vi "SRS865A_api -- V2.vi"(4 "Oscillator (0)":u16, 6 "delay-circle(msec)":i64, 7 "MFLI frontend action":T1=enum."open", 8 "Error In":errorcluster, 10 "Freq IN (Hz)":dbl=40000.0 format="%#_13g", 11 "SRS865 visa":refnum<visa-resource-name>="GPIB0::4::INSTR") -> (0 "Error Out":errorcluster={"status"=TRUE, "code"=-1074003951, "source"="Stanford Research SR865.lvlib:Initialize.vi<ERR>\nThe ID Query failed.  This may mean that you selected the wrong instrument or your instrument did not respond.  You may also be using a model that is not officially supported by this driver.  If you are sure that you have selected the correct instrument and it is responding, try disabling the ID Query.\n\n\n<b>Complete call chain:</b>\r\n     Stanford Research SR865.lvlib:Initialize.vi\r\n     SRS865A_api -- V2.vi\r\n     SRS865A--reader--V2.vi"}, 1 "z out (V)":cdb, 2 "Freq out (Hz)":dbl format="%#_13g", 3 "SRS865 visa OUT":refnum<visa-resource-name>)   [LabVIEW 2017]
uses:
  MFLI frontend action.ctl
  <instrlib>/Zurich Instruments LabOne/Zurich Instruments LabOne.lvlib
  <instrlib>/Stanford Research SR865/Stanford Research SR865.lvlib
panel:
  out "output 1":i32
  in  "timeconstant (s)":dbl=0.006
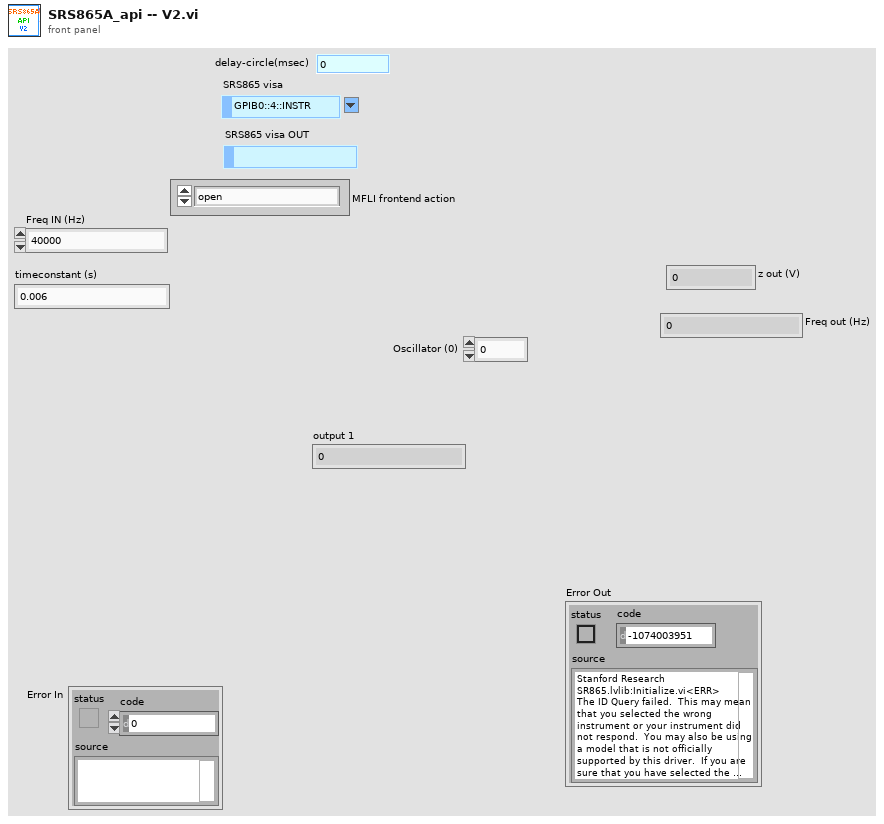
[diagram p1: front panel]
types:
  T1 = typedef "MFLI frontend action.ctl" = enum16{"read", "writeread", "open", "close", "write"}
  T2 = typedef "Zurich Instruments LabOne.lvlib/ziTypeHandle.ctl" = cluster{"handleValid":bool, "Conn":u64, "Path Prefix":string, "Handle":u64, "Connected":bool, "Clockbase(s)":dbl}
  T3 = cluster{"Timestamps (ticks)":u64, "X (Vrms)":dbl, "Y (Vrms)":dbl, "Osc Phase (deg)":dbl, "Freq (Hz)":dbl, "DIO":u32, "AuxIn0 (V)":dbl, "AuxIn1 (V)":dbl}
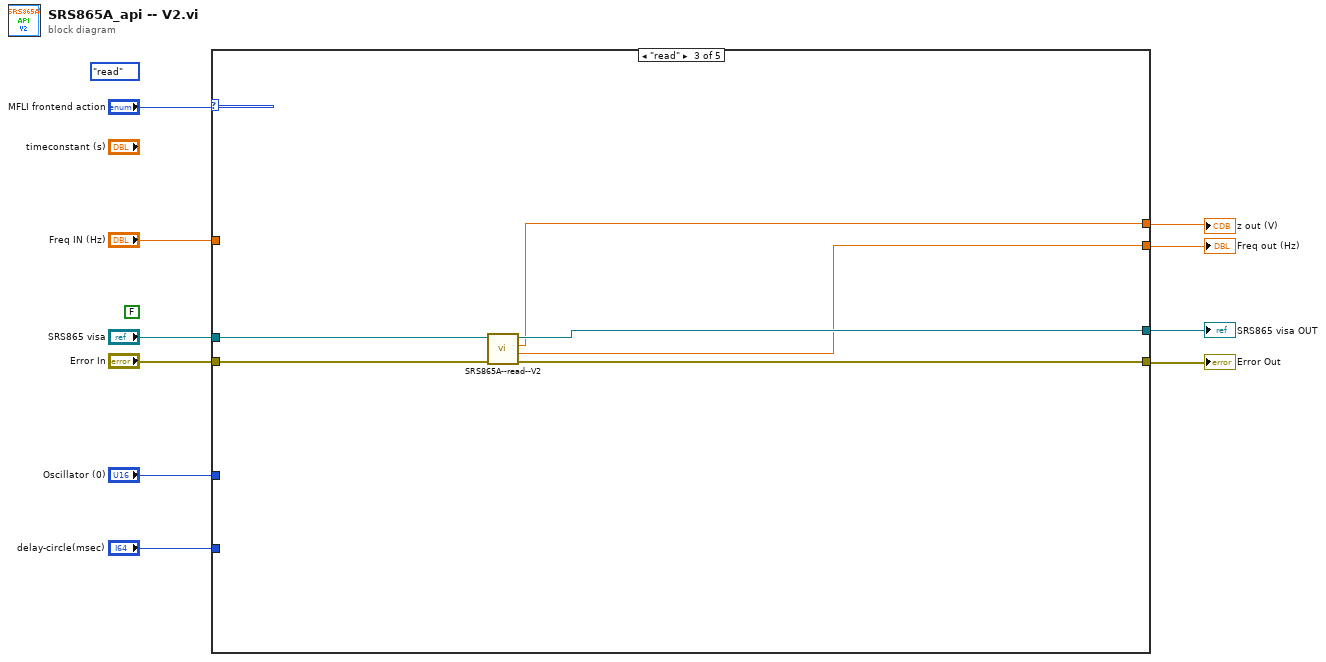
[diagram p0: block diagram]
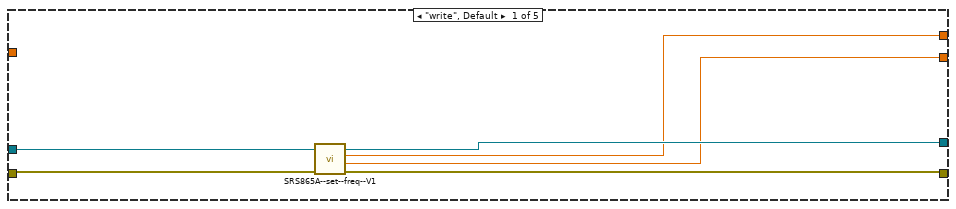
[diagram p2: hidden frame]
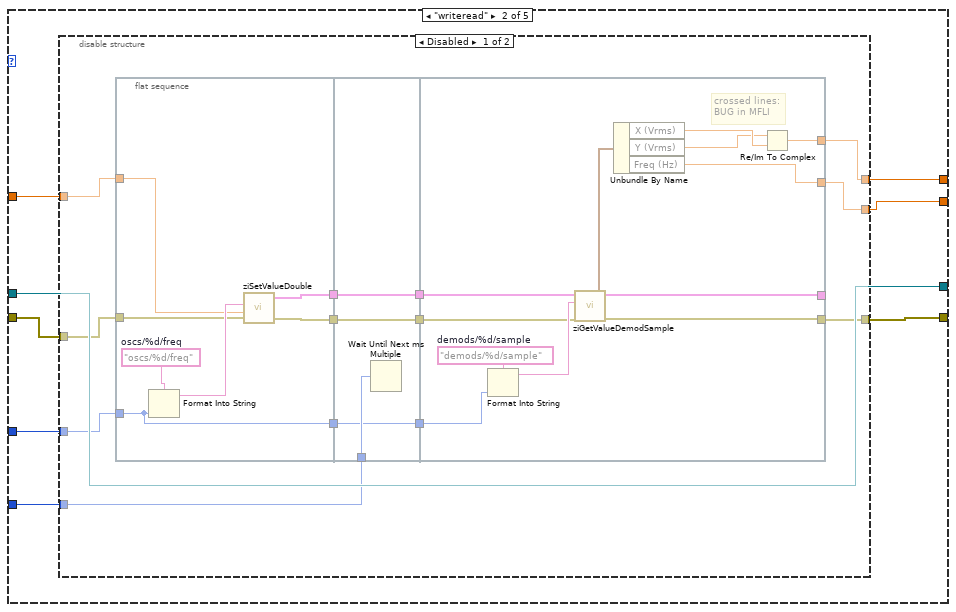
[diagram p3: hidden frame]
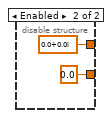
[diagram p4: hidden frame]
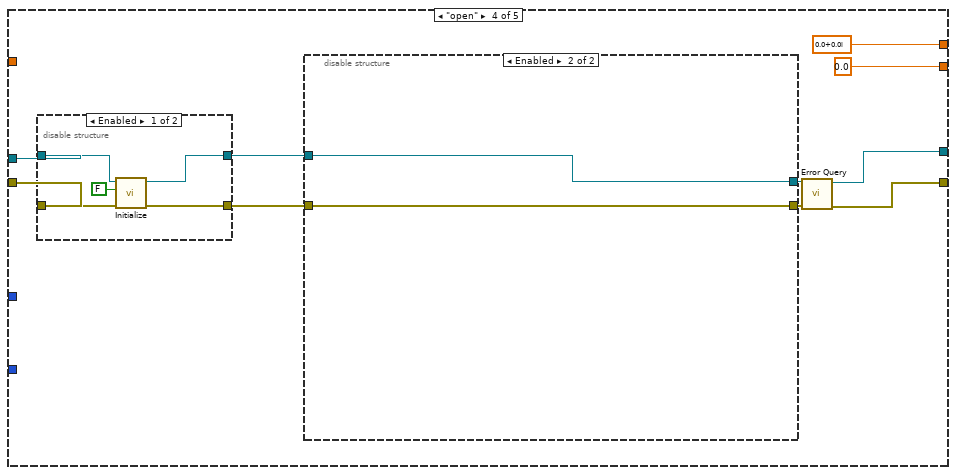
[diagram p5: hidden frame]
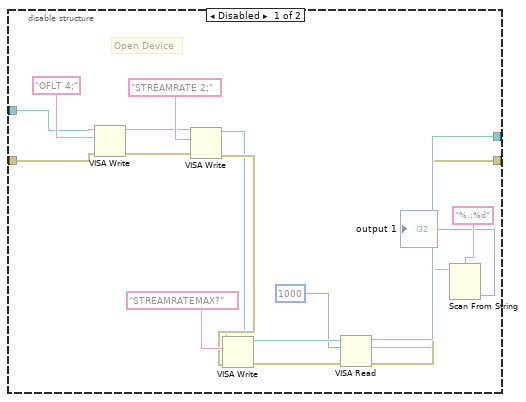
[diagram p6: hidden frame]
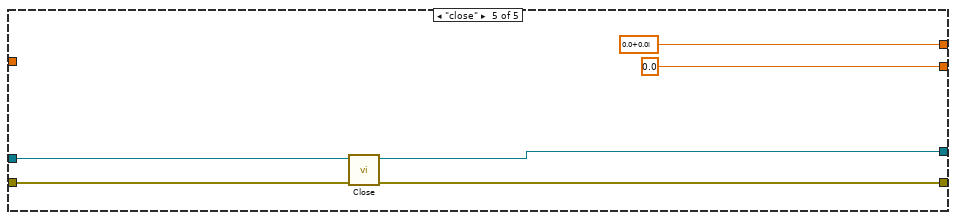
[diagram p8: hidden frame]
diagram:
  (unwired) MFLI_frontend_action."read" ("MFLI frontend action")
  (unwired) FALSE
  n1 = case shown="\"read\"" "MFLI frontend action" {
    tunnel: [w15 w16 w65 w71 w104] -> w2
    tunnel: [w13 w22 w64 w70 w107] -> w10
    tunnel: [w12 w17 w63 cdb 0.0+0.0i cdb 0.0+0.0i] -> w9
    tunnel: "SRS865 visa" -> [w15 w16 w66 w74 w104]
    tunnel: "Error In" -> [w14 w23 w67 w77 w108]
    tunnel: "Oscillator (0)" -> [_ w20 _ _ _]
    tunnel: [w11 w18 w62 0.0 ("Freq (Hz)") 0.0 ("Freq (Hz)")] -> w6
    tunnel: "Freq IN (Hz)" -> [_ w21 _ _ _]
    tunnel: "delay-circle(msec)" -> [_ w19 _ _ _]
    frame "write", Default {
      n2 = call "SRS865A--set--freq--V1.vi"("error in (no error)"=w14, "VISA resource name"=w15) -> ("error out"=w13:errorcluster, "freq out"=w11:dbl, "zi out (V)"=w12:cdb)  [unwired: 6 in, 1 out]
    }
    frame "writeread" {
      n3 = disable-structure shown="Disabled" {
        disable-tunnel: w23 -> [w30 _]
        disable-tunnel: [w29 _] -> w22
        disable-tunnel: w21 -> [w28 _]
        disable-tunnel: w20 -> [w27 _]
        disable-tunnel: w19 -> [w26 _]
        disable-tunnel: [w25 0.0 ("Freq (Hz)")] -> w18
        disable-tunnel: [w24 cdb 0.0+0.0i] -> w17
        frame Disabled {
          n4 = flat-sequence {
            tunnel: w30 -> [w41]
            tunnel: w28 -> [w38]
            tunnel: w27 -> [w37]
            tunnel: [w40] -> w36
            tunnel: [w39] -> w35
            tunnel: [w37] -> w34
            tunnel: w36 -> [w47]
            tunnel: w35 -> [w46]
            tunnel: [w47] -> w33
            tunnel: [w46] -> w32
            tunnel: w26 -> [w45]
            tunnel: w34 -> [w44]
            tunnel: [w44] -> w31
            tunnel: [w51] -> w29
            tunnel: [w49] -> _
            tunnel: w33 -> [w50]
            tunnel: w32 -> [w52]
            tunnel: [w54] -> w25
            tunnel: [w53] -> w24
            tunnel: w31 -> [w48]
            frame #0 {
              w43 = "oscs/%d/freq"  # oscs/%d/freq
              n5 = Format Into String(format string=w43, w37) -> (resulting string=w42:string)  [unwired: 2 in, 1 out]
              n6 = call <instrlib>:"ziSetValueDouble.vi"("Error In"=w41, "Value"=w38, "Path"=w42) -> ("Error Out"=w39:errorcluster, "Handle Out"=w40:T2)  [unwired: 2 in]
            }
            frame #1 {
              n7 = Wait Until Next ms Multiple(millisecond multiple=w45) -> ()  [unwired: 1 out]
            }
            frame #2 {
              w58 = "demods/%d/sample"  # demods/%d/sample
              # "crossed lines:\nBUG in MFLI"
              n8 = Format Into String(format string=w58, w48) -> (resulting string=w59:string)  [unwired: 2 in, 1 out]
              n9 = call <instrlib>:"ziGetValueDemodSample.vi"("error in"=w52, "Path"=w59, "Handle In"=w50) -> ("error out"=w51:errorcluster, "Demod Sample Out"=w57:T3, "Handle Out"=w49:T2)  [unwired: 2 in]
              n10 = Unbundle By Name(w57) -> ("X (Vrms)"=w56:dbl, "Y (Vrms)"=w55:dbl, "Freq (Hz)"=w54:dbl)
              n11 = Re/Im To Complex(1:w56, 2:w55) -> (0:w53:cdb)
            }
          }
        }
        frame Enabled {
        }
      }
    }
    frame "read" {
      n12 = call "SRS865A--read--V2.vi"("error in (no error)"=w67, "VISA resource name"=w66) -> ("error out"=w64:errorcluster, "freq out"=w62:dbl, "zi out (V)"=w63:cdb, "VISA resource name out"=w65:refnum<visa-resource-name>)  [unwired: 6 in]
    }
    frame "open" {
      n13 = disable-structure shown="Enabled" {
        disable-tunnel: w77 -> [w101 w102]
        disable-tunnel: [w100 w103] -> w68
        disable-tunnel: [w99 w102] -> w69
        disable-tunnel: w74 -> [w98 w103]
        frame Enabled {
          n14 = call <instrlib>:"Initialize.vi"("error in (no error)"=w101, "ID Query (True)"=FALSE, "VISA resource name"=w98) -> ("error out"=w99:errorcluster, "VISA resource name out"=w100:refnum<visa-resource-name>)  [unwired: 7 in]
        }
        frame Disabled {
        }
      }
      n15 = disable-structure shown="Enabled" {
        disable-tunnel: [w91 w96] -> w73
        disable-tunnel: [w89 w95] -> w72
        disable-tunnel: w69 -> [w81 w95]
        disable-tunnel: w68 -> [w79 w96]
        frame Disabled {
          # "Open Device"
          n16 = VISA Write(VISA resource name=w79, write buffer="OFLT 4;", error in (no error)=w81) -> (VISA resource name out=w78:refnum<visa-resource-name>, error out=w80:errorcluster)  [unwired: 1 out]
          n17 = VISA Write(VISA resource name=w78, write buffer="STREAMRATE 2;", error in (no error)=w80) -> (VISA resource name out=w85:refnum<visa-resource-name>, error out=w86:errorcluster)  [unwired: 1 out]
          n18 = VISA Write(VISA resource name=w85, write buffer="STREAMRATEMAX?", error in (no error)=w86) -> (VISA resource name out=w92:refnum<visa-resource-name>, error out=w90:errorcluster)  [unwired: 1 out]
          n19 = VISA Read(VISA resource name=w92, byte count=u32 1000, error in (no error)=w90) -> (VISA resource name out=w91:refnum<visa-resource-name>, read buffer=w88:string, error out=w89:errorcluster)  [unwired: 1 out]
          n20 = Scan From String(format string="%.;%d", input string=w88) -> (output 1=→"output 1":i32)  [unwired: 3 in, 3 out]
        }
        frame Enabled {
        }
      }
      n21 = call <instrlib>:"Error Query.vi"("error in (no error)"=w72, "VISA resource name"=w73) -> ("error out"=w70:errorcluster, "VISA resource name out"=w71:refnum<visa-resource-name>)  [unwired: 7 in, 1 out]
    }
    frame "close" {
      n22 = call <instrlib>:"Close.vi"("error in (no error)"=w108, "VISA resource name"=w104) -> ("error out"=w107:errorcluster)  [unwired: 9 in]
    }
  }
  "Error Out" <- w10
  "z out (V)" <- w9
  "Freq out (Hz)" <- w6
  "SRS865 visa OUT" <- w2
